vi "Beat Sound Octave.vi"() -> ()   [LabVIEW 2021]
doc: "This VI illustrates how to generate and play sine, square, sawtooth and triangle waveforms. You can change the frequency and type of the waveform generated as it plays continuously."
uses:
  <vilib>/sound2/lvsound2.llb/Sampling Mode.ctl
  <vilib>/sound2/lvsound2.llb/Sound Data Format.ctl
  <vilib>/sound2/lvsound2.llb/Sound Output Set Volume (Single).vi
  <vilib>/sound2/lvsound2.llb/Sound Output Write (DBL Single).vi
  <vilib>/measure/NI_MABase.lvlib
panel:
  in  "Frequencies [Hz]":dbl[](array[slide])=[440.0, 880.0] min=300.0 max=1000.0 step=1.0 scale=400.0..1000.0
  in  "Volume":dbl(slide)=21.338912133891213 scale=0.0..100.0
  out "Generated Sound":waveform(dbl)[](graph)=[{"t0"=timestamp(9.993764172335602 s since 1904-01-01), "dt"=2.2675736961451248e-05, "Y"=array[2005 elements]}, {"t0"=timestamp(9.993764172335602 s since 1904-01-01), "dt"=2.2675736961451248e-05, "Y"=array[2005 elements]}, {"t0"=timestamp(9.993764172335602 s since 1904-01-01), "dt"=2.2675736961451248e-05, "Y"=array[2005 elements]}]
  in  "Stop":bool
  # "Beat Tone Demo"
  # "McClellan et al., DSP First 3-4 Periodic Waveforms"
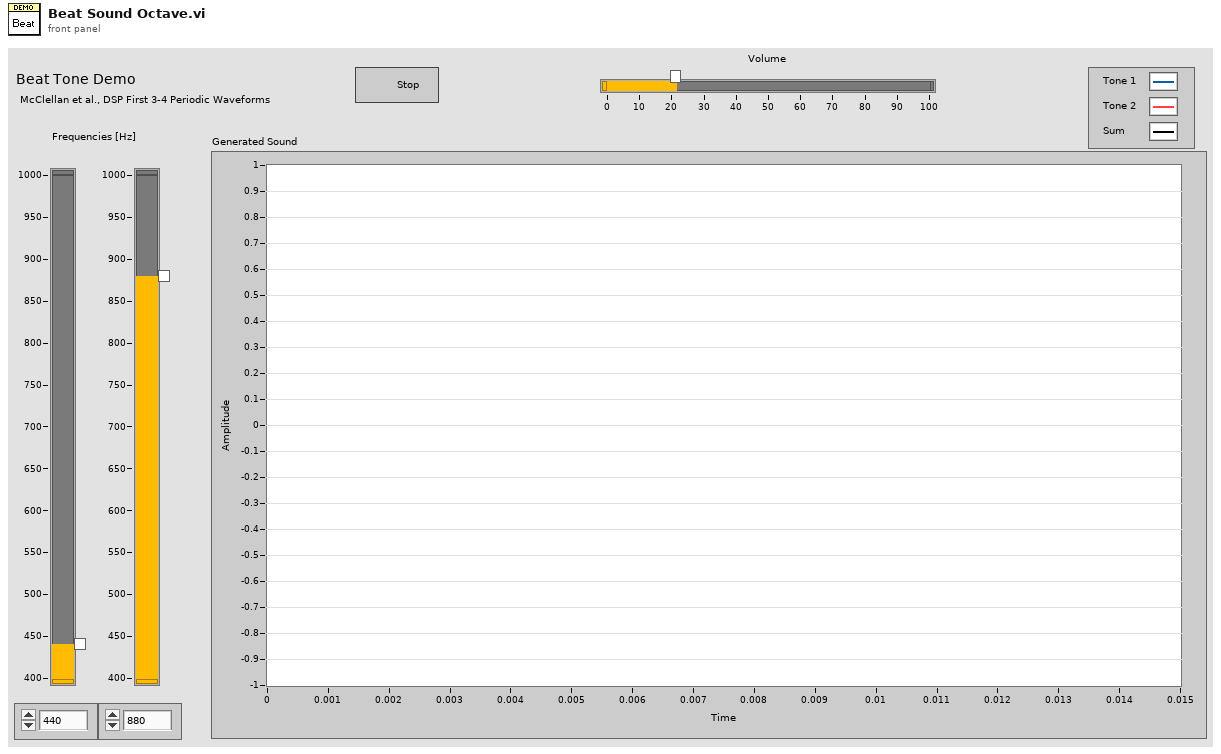
[diagram p1: front panel]
types:
  T1 = typedef "Sound Data Format.ctl" = cluster{"sample rate (S/s)":dbl, "number of channels":i32, "bits per sample":i32}
  T2 = typedef "Sampling Mode.ctl" = i32
  T3 = typedef "Sound Output Task ID.ctl" = u32
  T4 = enum16{"Sine Wave", "Triangle Wave", "Square Wave", "Sawtooth Wave"}
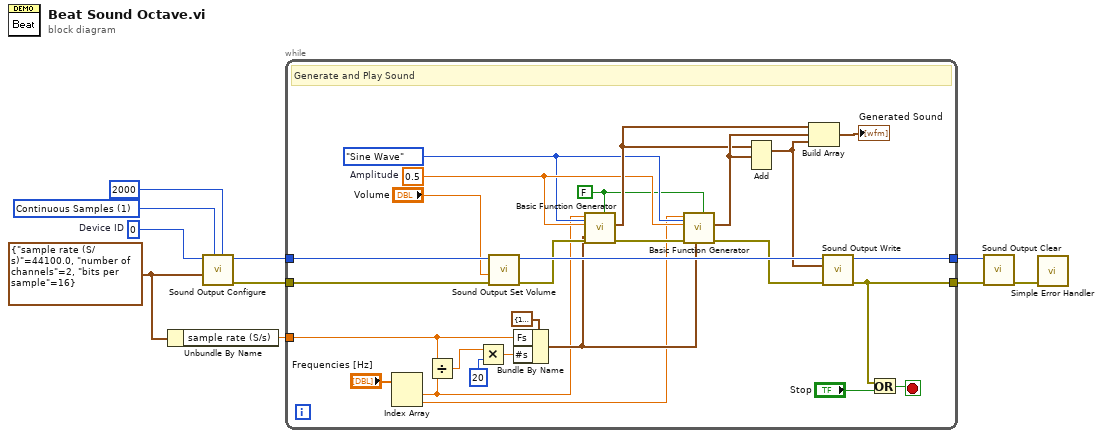
[diagram p0: block diagram]
diagram:
  w6 = u32 0  # Device ID
  w3 = T1 {"sample rate (S/s)"=44100.0, "number of channels"=2, "bits per sample"=16} ("Sound Format")
  w1 = T2 1 items=["Finite Samples", "Continuous Samples"] ("sample mode")
  n1 = Unbundle By Name(w3) -> ("sample rate (S/s)"=w4:dbl)
  n2 = call <vilib>:"Sound Output Configure.vi"("number of samples/ch"=2000 ("Number of Samples/ch"), "sample mode"=w1, "sound format"=w3, "device ID"=w6) -> ("error out"=w10:errorcluster, "task ID"=w9:T3)  [unwired: 6 in]
  n3 = while {
    tunnel: w9 -> [w32]
    tunnel: [w37] -> w7
    tunnel: w10 -> [w34]
    tunnel: [w30] -> w8
    tunnel: w4 -> [w16]
    stop <- w35 stop-if-true
    w18 = FALSE ("reset signal")
    w21 = 0.5  # Amplitude
    w20 = T4."Sine Wave" ("signal type")
    # "Generate and Play Sound"
    n4 = Index Array(array="Frequencies [Hz]") -> (element #1=w12:dbl, element #2=w13:dbl)  [unwired: 2 in]
    n5 = Divide(x=w16, y=w12) -> (x/y=w14:dbl)
    n6 = Multiply(x=w14, y=20) -> (x*y=w11:dbl)
    n7 = call-poly <vilib>:"Sound Output Set Volume.vi"("error in (no error)"=w34, "volume"="Volume", "task ID"=w32) -> ("error out"=w28:errorcluster, "task ID out"=w33:T3)  [unwired: 7 in]
    n8 = Bundle By Name(cluster=cluster{"Fs":dbl, "#s":dbl} {"Fs"=1000.0, "#s"=1000.0} ("sampling info"), "Fs"=w16, "#s"=w11) -> (w25:cluster{"Fs":dbl, "#s":dbl})
    n9 = call <vilib>:"Basic Function Generator.vi"("reset signal"=w18, "sampling info"=w25, "signal type"=w20, "error in (no error)"=w28, "amplitude"=w21, "frequency"=w12) -> ("error out"=w19:errorcluster, "signal out"=w23:waveform(dbl))  [unwired: 3 in, 1 out]
    n10 = call <vilib>:"Basic Function Generator.vi"("reset signal"=w18, "sampling info"=w25, "signal type"=w20, "error in (no error)"=w19, "amplitude"=w21, "frequency"=w13) -> ("error out"=w26:errorcluster, "signal out"=w24:waveform(dbl))  [unwired: 3 in, 1 out]
    n11 = Add(1:w24, 2:w23) -> (0:w22:waveform(dbl))  [unwired: 1 in, 1 out]
    n12 = Build Array(w23, w24, w22) -> (→"Generated Sound":waveform(dbl)[])
    n13 = call-poly <vilib>:"Sound Output Write.vi"("error in (no error)"=w26, "data"=w22, "task ID"=w33) -> ("error out"=w30:errorcluster, "task ID out"=w37:T3)  [unwired: 7 in]
    n14 = Or(x=w30, y="Stop") -> (x .or. y?=w35:bool)
  }
  n15 = call <vilib>:"Sound Output Clear.vi"("error in (no error)"=w8, "task ID"=w7) -> ("error out"=w5:errorcluster)  [unwired: 9 in]
  n16 = call <vilib>:"Simple Error Handler.vi"("error in (no error)"=w5) -> ()  [unwired: 4 in, 5 out]
